vi "Dashboard Main.vi"() -> ()   [LabVIEW 2015]
uses:
  <vilib>/Utility/miscctls.llb/LVRowAndColumnTypeDef.ctl
  <vilib>/event_ctls.llb/eventvkey.ctl
  <vilib>/Rock Robotics/WPI/Dashboard/WPI_DashboardLogging Global.vi
  <vilib>/Utility/config.llb/Write Key (String).vi
  <vilib>/Utility/config.llb/Write Key (I32).vi
  <vilib>/Utility/config.llb/NI_LVConfig.lvlib
  <vilib>/vision/NI_Vision_Development_Module.lvlib
panel:
  in  "TCP":refnum<k5>
  in  "Rec Mode":enum32{"Stop", "Record", "Playback"}(radio)
  in  "Vision":u16(ring)=2 items=["Camera Off", "USB Camera SW", "USB Camera HW", "IP Camera"]
  out "Camera IP":string
  out "Image Message":string="Timeout in Camera Communications"
  in  "Dashboard Tab":T1(tab)
  in  "Two Ball Auto":bool=TRUE
  in  "Defense Selector":u16(ring) items=["Low Bar", "Ramparts", "Moat", "Rock Wall", "Rough Terrain", "Portcullis", "Cheval de Frise", "Drawbridge", "Sally Port"]
  out "Right 2 Current":dbl
  out "Right 1 Current":dbl
  out "Left 2 Current":dbl
  out "Left 1 Current":dbl
  in  "ManipulatorSelector":u16(ring) items=["Portcullis", "Cheval"]
  out "Flip Image":bool
  in  "OK Button":bool
  in  "Position Selector":u16(ring) items=["Far Left", "Pos 2", "Pos 3", "Pos 4", "Far Right"]
  out "NT Connection":bool
  in  "Camera Settings":T2={"Frame Rate"=14, "Compression"=30, "Size"=0} {"Frame Rate" scale=1.0..30.0; "Size" items=["640x480", "320x240", "160x120"]}
  out "Gyro":dbl(knob) scale=0.0..360.0
  out "JS1 Z":dbl(slide) scale=-1.0..1.0 scale format="%#_2e"
  out "JS1 Graph":cluster{"X":dbl, "Y":dbl}[](graph)
  out "JS1 Buttons":T3
  out "JS2 Z":dbl(slide) scale=-1.0..1.0 scale format="%#_2e"
  out "JS2 Graph":cluster{"X":dbl, "Y":dbl}[](graph)
  out "JS2 Buttons":T3
  out "Mode":T4(ring)=enum."Disconnected"
  in  "DB Camera Config":bool
  out "fps":dbl format="%#.1g"
  out "Mbps":dbl=9.6e-05 format="%#.1g"
  out "Mbps LED":bool
  out "Auto Target Enabled":bool
  out "On Target":bool
  out "Ball In Roller":bool
  in  "DB/String 9":string
  in  "DB/String 8":string
  in  "DB/String 7":string
  in  "DB/String 6":string
  in  "DB/String 5":string
  in  "DB/String 4":string
  in  "DB/String 3":string
  in  "DB/String 2":string
  in  "DB/String 1":string
  in  "DB/String 0":string
  in  "DB/Slider 0":dbl(slide) scale=0.0..5.0
  in  "DB/Slider 1":dbl(slide) scale=0.0..5.0
  in  "DB/Slider 2":dbl(slide) scale=0.0..5.0
  in  "DB/Slider 3":dbl(slide) scale=0.0..5.0
  out "DB/LED 3":bool
  out "DB/LED 2":bool
  out "DB/LED 1":bool
  out "DB/LED 0":bool
  in  "DB/Button 3":bool
  in  "DB/Button 2":bool
  in  "DB/Button 1":bool
  in  "DB/Button 0":bool caption="New Name"
  in  "Test Slider":dbl(slide) scale=0.0..100.0 scale format="%#_3g"
  in  "On/Off":bool caption="Solenoid"
  in  "Test Name":u16(ring) items=["Select the test to run..."]
  in  "Test Tree":string(tree)
  in  "Motor":cluster{"Value":dbl, "Enable":bool} {"Value" scale=-1.0..1.0 scale format="%#_3g"}
  out "Progress":T5 {"Test Progress" scale=0.0..100.0}
  in  "Rev/Fwd":cluster{"Forward":bool, "Reverse":bool}
  in  "Test Ring":u16(ring) items=["Monochrome", "Color"]
  out "Cmd Status":string
  in  "Execute Command":bool
  in  "Command Params":string[][](table)
  in  "Command Selection":i32(listbox)
  in  "CheckList":i32(listbox)
  out "Tree":string(tree)
  out "Camera Image":T6(plugin-control)
  out "Background":bool
  # "Left"
  # "Front"
  # "Right"
  # "This tab is a great place for autonomous settings and robot-specific values.\nPlace controls and indicators inside this tab and match name to\nDashboard Variables on robot. You can also delete this comment."
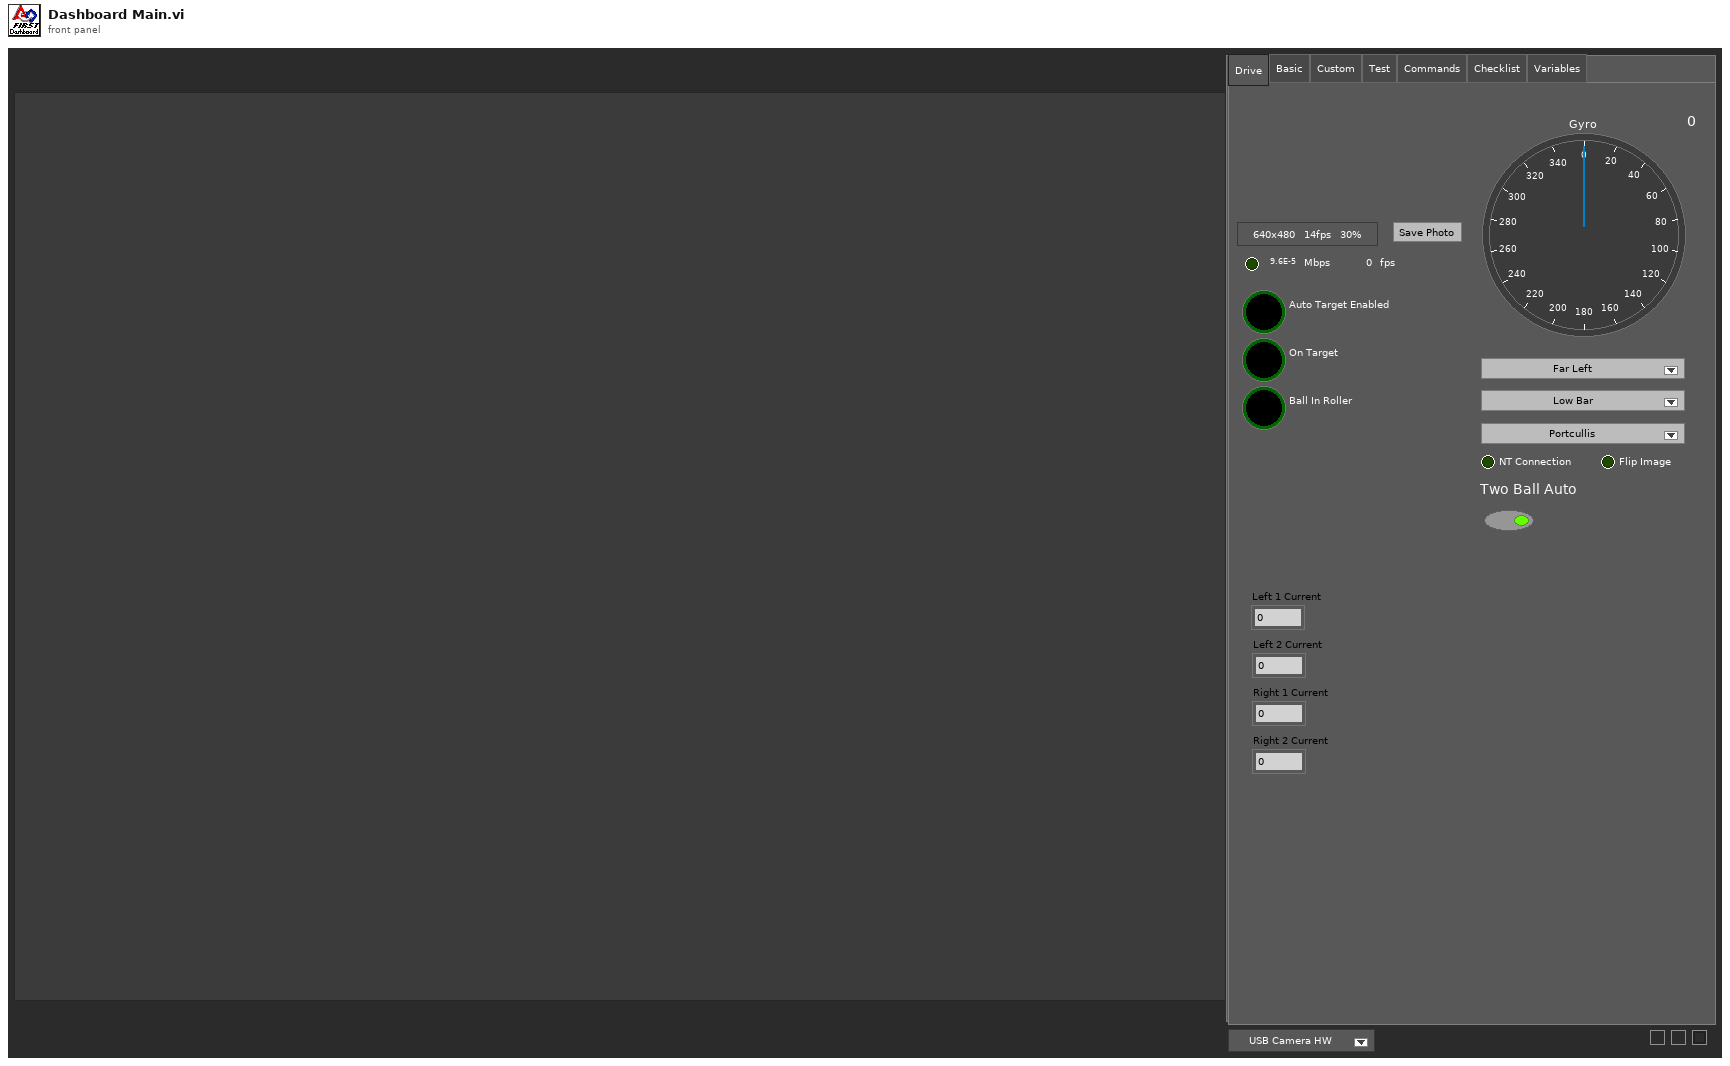
[diagram p1: front panel]
types:
  T1 = enum32{"Drive", "Basic", "Custom", "Test", "Commands", "Checklist", "Variables"}
  T2 = cluster{"Frame Rate":i32, "Compression":i32, "Size":u16}
  T3 = cluster{bool, bool, bool, bool, bool, bool, bool, bool, bool, bool, bool, bool}
  T4 = enum8{"Tele-Op Disabled", "Tele-Op Enabled", "Auto Disabled", "Auto Enabled", "Test Disabled", "Test Enabled", "Disconnected", "No Code", "E-Stop"}
  T5 = cluster{"Test Progress":u8, "Test Progress Text":string}
  T6 = typedef "IMAQ Image.ctl" = refnum<image>
  T7 = typedef "Image Type" = u32
  T8 = cluster{"IDs":cluster{"RPC field ID":u16, "Unique ID":u16}, "String":string}
  T9 = enum32{"Drive", "Basic", "Custom", "Test", "Checklist", "Variables"}
  T10 = cluster{"Camera Image":refnum<vi>, "Dashboard Tab":refnum<vi>, "Background":refnum<vi>, "Vision":refnum<vi>, "Rec Mode":refnum<vi>, "Test Slider":refnum<vi>, "On/Off ":refnum<vi>, "Test Ring":refnum<vi>, "Rev/Fwd":refnum<vi>, "Test Name":refnum<vi>, "Motor":refnum<vi>, "Progress":refnum<vi>, "CheckList":refnum<vi>, "Tree":refnum<vi>, "Test Tree":refnum<vi>, "Command Params":refnum<vi>, "Command Selection":refnum<vi>, "Execute Command":refnum<vi>, "Cmd Status":refnum<vi>}
  T11 = typedef "NI_LVConfig.lvlib/Config Data RefNum.ctl" = refnum<k1>
  T12 = cluster{"Operation":enum16{"Update", "Clear"}, "Color Box":u32}[]
  T13 = typedef "eventvkey.ctl" = enum16{"ASCII", "Enter", "Return", "Shift", "Ctrl", "Alt", "Cmd", "Opt", "Caps", "NumLock", "Clear", "Break", "Up", "Down", "Left", "Right", "Insert", "Delete", "Home", "End", "PageUp", "PageDown", "Escape", "Help", "Pause", "ScrollLock", "F1", "F2", "F3", "F4", "F5", "F6", "F7", "F8", "F9", "F10", "F11", "F12", "F13", "F14", "F15", "F16", "F17", "F18", "F19", "F20", "F21", "F22", "F23", "F24", "Play", "VolumeUp", "VolumeDown", "Mute", "Two Byte Char"}
  T14 = cluster{"Image Size":bool, "Image Type":bool, "Pixel Value":bool, "ROI Information":bool, "Zoom Factor":bool}
  T15 = enum8{"Enabled", "Disabled", "Disabled and Grayed Out"}
  T16 = cluster{"Operation":enum16{"Update", "Clear"}, "Color Box":u32}
  T17 = typedef "LVRowAndColumnTypeDef.ctl" = cluster{"Row":i32, "Column":i32}
  T18 = cluster{"Shift":bool, "Ctrl":bool, "Alt":bool, "Cmd":bool, "Opt":bool}
  T19 = cluster{"Error Strings":string, "Disable Counts":cluster{u16, u16}, "Rail Faults":cluster{u16, u16, u16}, "Robot IP":string, "DB Mode":u8, "Event Info":cluster{"Name":string, "Type":u8, "Number":u16, "Replay":u8}, "Camera Addr":string}
  T20 = cluster{"Storage":cluster{"Disk Free":u64, "RAM Block":u32, "RAM free":u32}, "CPU Utilization":cluster{"CPU % ISR":sgl, "CPU % Time Crit":sgl, "CPU % Timed Str":sgl, "CPU % High":sgl, "CPU % Above":sgl, "CPU % Normal":sgl, "CPU % Low":sgl}, "CAN":cluster{"% Bus Utilization":sgl, "Bus Off Cnt":u32, "TX_FIFO Full Cnt":u32, "Receive Error Cnt":u8, "Transmit Error Cnt":u8}, "HID":cluster{"HID Outputs":u32, "Rumble Low":u16, "Rumble High":u16}[]}
  T21 = cluster{"Status bits":cluster{"Test Mode":bool, "Autonomous":bool, "Enabled":bool, "Code Start":bool, "Brownout":bool, "Reserved 2":bool, "Reserved 3":bool, "E-Stop":bool}, "Code Trace":cluster{"Disabled":bool, "TeleOp":bool, "Auto":bool, "Test":bool}, "Controller Type":enum16{"unknown", "cRIO", "roboRio"}, "Code?":enum16{"unknown", "noCode", "code"}, "Battery V":dbl}
  T22 = cluster{"Control Bits":cluster{"TestMode":bool, "Autonomous":bool, "Enabled":bool, "FMS Present":bool, bool, bool, bool, "E-Stop":bool}, "Team Station ":u8, "Countdown":sgl, "Joystick Values":cluster{"Axes":dbl[], "Buttons":bool[], "POVs":i16[]}[]}
  T23 = cluster{"Axes":dbl[], "Buttons":bool[], "POVs":i16[]}[]
  T24 = cluster{"Axes":dbl[], "Buttons":bool[], "POVs":i16[]}
  T25 = cluster{"Buttons[0]":bool, "Buttons[1]":bool, "Buttons[2]":bool, "Buttons[3]":bool, "Buttons[4]":bool, "Buttons[5]":bool, "Buttons[6]":bool, "Buttons[7]":bool, "Buttons[8]":bool, "Buttons[9]":bool, "Buttons[10]":bool, "Buttons[11]":bool}
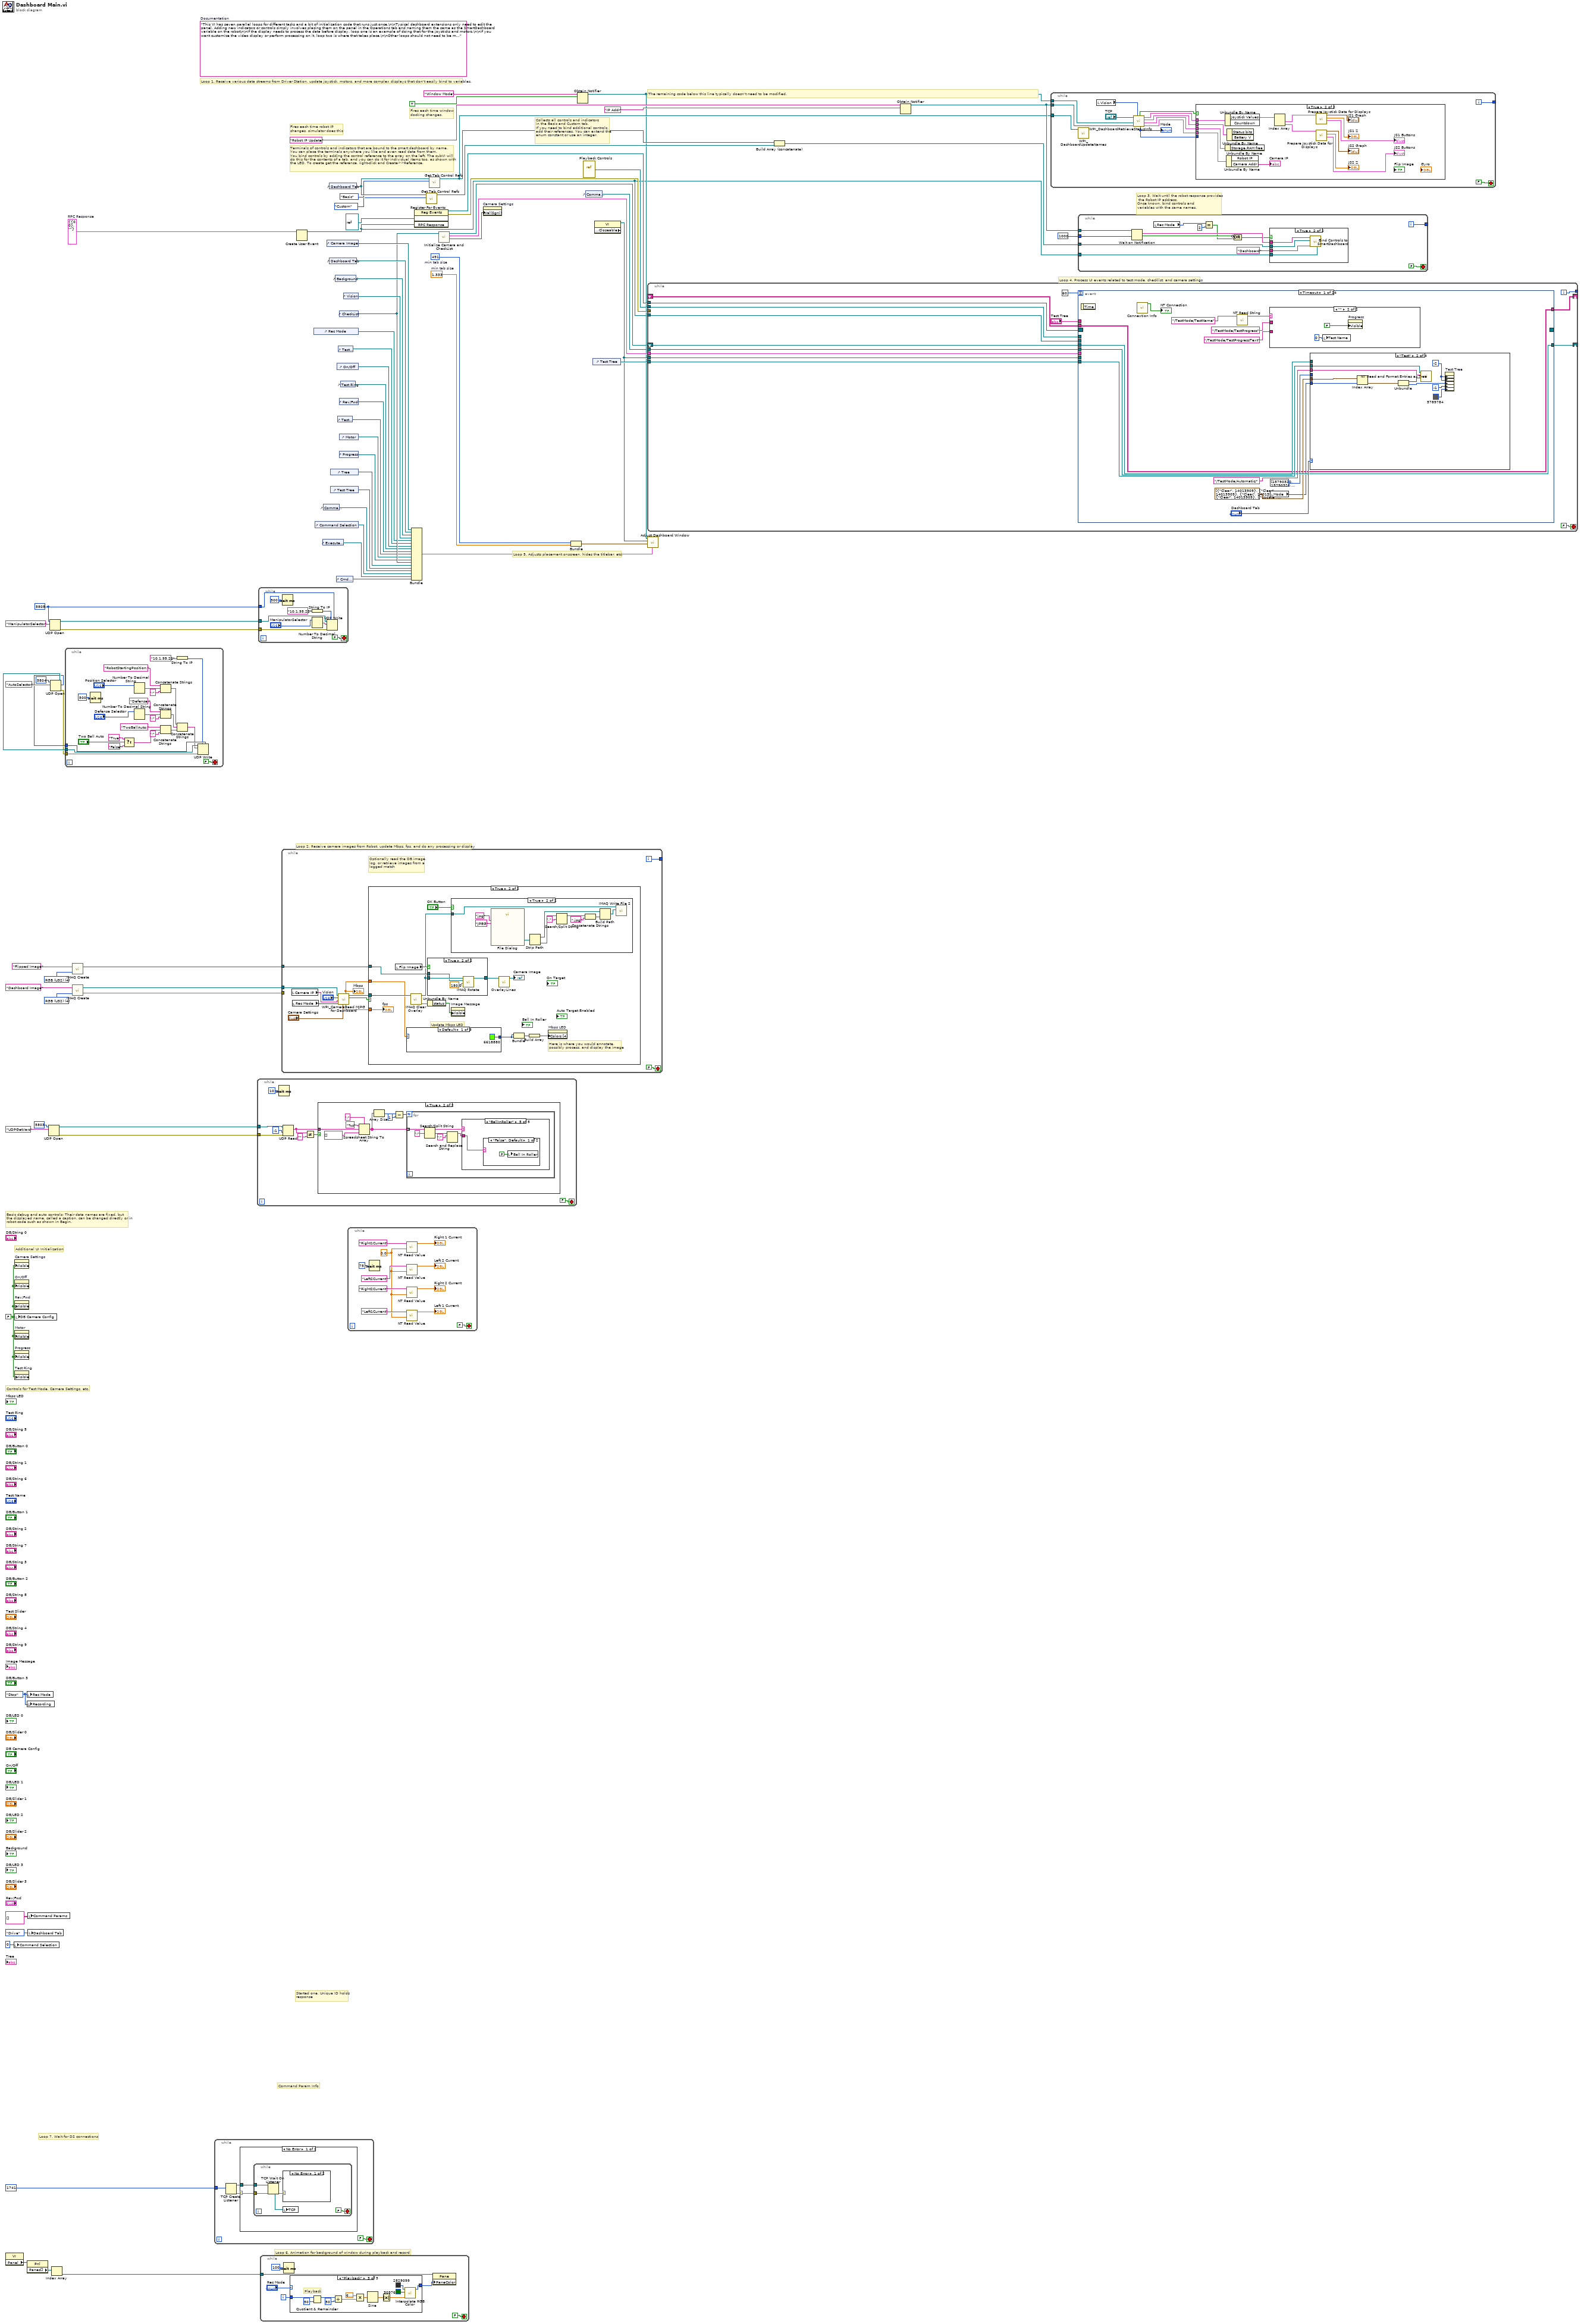
[diagram p0: block diagram]
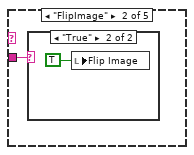
[diagram p4: hidden frame]
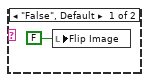
[diagram p5: hidden frame]
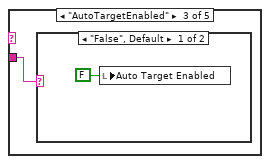
[diagram p6: hidden frame]
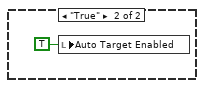
[diagram p7: hidden frame]
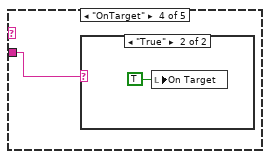
[diagram p8: hidden frame]
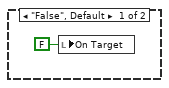
[diagram p9: hidden frame]
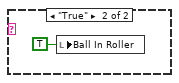
[diagram p10: hidden frame]
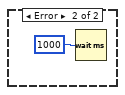
[diagram p11: hidden frame]
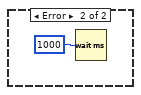
[diagram p12: hidden frame]
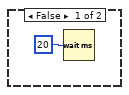
[diagram p13: hidden frame]
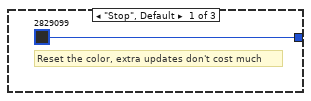
[diagram p14: hidden frame]
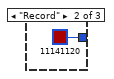
[diagram p15: hidden frame]
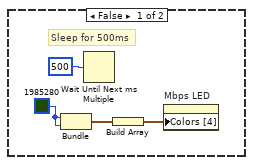
[diagram p17: hidden frame]
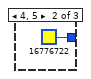
[diagram p20: hidden frame]
diagram:
  w1 = u16 5805 ("port")
  w7 = T7 4 items=["Grayscale (U8)", "Grayscale (I16)", "Grayscale (SGL)", "Complex (CSG)", "RGB (U32)", "HSL (U32)", "RGB (U64)"] ("Image Type")
  w23 = T8 {"IDs"={"RPC field ID"=0, "Unique ID"=0}, "String"=""}  # RPC Response
  w49 = 491  # min tab size
  w48 = 1.333  # min tab size
  w57 = enum32{"Stop", "Record", "Playback"}."Stop" ("Rec Mode")
  w31 = FALSE ("Visible")
  (unwired) "This VI has seven parallel loops for different tasks and a bit of initialization code that runs just once.\n\nTypical dashboard extensions only need to edit the panel. Adding new indicators or controls simply involves placing them on the panel in the Operations tab and naming them the same as the SmartDashboard variable on the robot\n\nIf the display needs to process the data before display, loop one is an example of doing that for the joysticks and motors.\n\nIf you want customize the video display or perform processing on it, loop two is where that takes place.\n\nOther loops should not need to be modified. They are pretty standard, and document the task they perform."  # Documentation
  w77 = T7 4 items=["Grayscale (U8)", "Grayscale (I16)", "Grayscale (SGL)", "Complex (CSG)", "RGB (U32)", "HSL (U32)", "RGB (U64)"] ("Image Type")
  # "Command Param Info"
  # "Started one, Unique ID holds\nresponse"
  # "Loop 7. Wait for DS connections"
  # "Basic debug and auto controls: Their data names are fixed, but\nthe displayed name, called a caption, can be changed directly or in\nrobot code such as shown in Begin."
  # "Controls for Test Mode, Camera Settings, etc."
  # "Additional UI Initialization"
  # "Loop 6. Animation for background of window during playback and record"
  # "Fires each time robot IP\nchanges, simulator does this"
  # "Fires each time window\ndocking changes."
  # "Collects all controls and indicators\nin the Basic and Custom tab.\nIf you need to bind additional controls,\nadd their references. You can extend the\nenum constant or use an integer."
  # "The remaining code below this line typically doesn't need to be modified."
  # "Loop 4. Process UI events related to test mode, checklist, and camera settings"
  # "Terminals of controls and indicators that are bound to the smart dashboard by name.\nYou can place the terminals anywhere you like and even read data from them.\nYou bind controls by adding the control reference to the array on the left. The subVI will\ndo this for the contents of a tab, and you can do it for individual items too, as shown with\nthe LED. To create get the reference, right-click and Create>>Reference."
  # "Loop 3. Wait until the robot response provides\n the Robot IP address.\nOnce known, bind controls and\nvariables with the same names."
  # "Loop 5. Adjusts placement onscreen, hides the titlebar, etc."
  # "Loop 1. Receive various data streams from Driver Station, update joystick, motors, and more complex displays that don't easily bind to variables."
  # "Loop 2. Receive camera images from Robot, update Mbps, fps, and do any processing or display"
  n1 = property class="VI"() -> ("Panel"=w64:refnum<vi>)  [unwired: 2 in, 2 out]
  n2 = local write "Command Selection"(u16 0 ("milliseconds to wait")) -> ()
  n3 = property on="Camera Settings" class="Clust (strict)"("Visible"=w31) -> ()  [unwired: 2 in, 2 out]
  n4 = property on="On/Off" class="Bool (strict)"("Visible"=w31) -> ()  [unwired: 2 in, 2 out]
  n5 = property on="Rev/Fwd" class="Clust (strict)"("Visible"=w31) -> ()  [unwired: 2 in, 2 out]
  n6 = local write "DB Camera Config"(w31) -> ()
  n7 = property on="Motor" class="Clust (strict)"("Visible"=w31) -> ()  [unwired: 2 in, 2 out]
  n8 = property on="Progress" class="Clust (strict)"("Visible"=w31) -> ()  [unwired: 2 in, 2 out]
  n9 = property on="Test Ring" class="Ring (strict)"("Visible"=w31) -> ()  [unwired: 2 in, 2 out]
  n10 = local write "Rec Mode"(w57) -> ()
  n11 = global write "WPI_DashboardLogging Global.vi" "Recording"(w57) -> ()
  n12 = property class="Pnl"(reference=w64) -> ("Panes[]"=w65:refnum<vi>[])  [unwired: 1 in, 2 out]
  n13 = local write "Command Params"(string[][] [] ("Command Params")) -> ()
  n14 = local write "Dashboard Tab"(T1."Drive" ("Dashboard Tab")) -> ()
  n15 = UDP Open(10:"UDPGetVars" ("service name"), 11:u16 5803 ("port")) -> (port=w11:refnum<k16>, 0:w10:errorcluster)  [unwired: 3 in, 1 out]
  n16 = UDP Open(10:"ManipulatorSelector" ("service name"), 11:w1) -> (port=w4:refnum<k16>, 0:w3:errorcluster)  [unwired: 3 in, 1 out]
  n17 = UDP Open(10:"AutoSelector" ("service name"), 11:u16 5804 ("port")) -> (port=w14:refnum<k16>, 0:w12:errorcluster, 2:w13:u16)  [unwired: 3 in]
  n18 = Index Array(array=w65) -> (element=w63:refnum<vi>)  [unwired: 1 in]
  n19 = while {
    tunnel: w14 -> [w100]
    tunnel: w13 -> [w99]
    tunnel: w12 -> [w96]
    stop <- FALSE stop-if-true
    n20 = Wait (ms)(milliseconds to wait=u32 500) -> ()  [unwired: 1 out]
    n21 = Select(t="True" ("string"), s="Two Ball Auto", f="False" ("string")) -> (s? t:f=w81:string)
    n22 = Number To Decimal String(number="Position Selector") -> (decimal integer string=w94:string)  [unwired: 1 in]
    n23 = Number To Decimal String(number="Defense Selector") -> (decimal integer string=w90:string)  [unwired: 1 in]
    n24 = Concatenate Strings("RobotStartingPosition:" ("string"), w94, ";" ("string")) -> (w85:string)
    n25 = Concatenate Strings("Defense:" ("string"), w90, ";" ("string")) -> (w84:string)
    n26 = Concatenate Strings("TwoBallAuto:" ("string"), w81, ";" ("string")) -> (w82:string)
    n27 = String To IP(1:"10.1.95.22") -> (0:w97:u32)
    n28 = Concatenate Strings(w85, w84, w82) -> (w83:string)
    n29 = UDP Write(address=w97, port or service name=w99, connection ID=w100, data in=w83, 8:w96) -> ()  [unwired: 1 in, 2 out]
  }
  n30 = call "IMAQ Create"("Image Name"="Flipped Image", "Image Type"=w7) -> ("New Image"=w5:T6)  [unwired: 2 in, 2 out]
  n31 = call "IMAQ Create"("Image Name"="Dashboard Image", "Image Type"=w77) -> ("New Image"=w75:T6, "error out"=w74:errorcluster)  [unwired: 2 in, 1 out]
  n32 = while {
    tunnel: u16 1741 ("timeout ms (25000)") -> [w104]
    stop <- FALSE stop-if-true
    n33 = TCP Create Listener(10:w104) -> (0:w103:errorcluster, 3:w105:refnum<k5>)  [unwired: 4 in, 1 out]
    n34 = case shown="No Error" w103 {
      selector: w103 -> [w107 _]
      tunnel: w105 -> [w108 _]
      frame No Error {
        n35 = while {
          tunnel: w108 -> [w111]
          tunnel: w107 -> [w110]
          stop <- FALSE stop-if-true
          n36 = TCP Wait On Listener(8:w110, 11:w111) -> (0:w112:errorcluster, 4:w113:refnum<k5>)  [unwired: 2 in, 3 out]
          n37 = case shown="No Error" w112 {
            frame No Error {
            }
            frame Error {
              n38 = Wait (ms)(milliseconds to wait=u32 1000) -> ()  [unwired: 1 out]
            }
          }
          n39 = local write "TCP"(w113) -> ()
        }
      }
      frame Error {
        n40 = Wait (ms)(milliseconds to wait=u32 1000) -> ()  [unwired: 1 out]
      }
    }
  }
  n41 = while {
    tunnel: w11 -> [w120]
    tunnel: w10 -> [w119]
    stop <- FALSE stop-if-true
    n42 = Wait (ms)(milliseconds to wait=u32 10) -> ()  [unwired: 1 out]
    n43 = UDP Read(connection ID=w120, timeout ms (25000)=-1, 8:w119) -> (data out=w116:string)  [unwired: 1 in, 4 out]
    n44 = Not Equal?(x=w116, y="") -> (x != y?=w117:bool)
    n45 = case shown="True" w117 {
      tunnel: w116 -> [_ w131]
      frame False {
      }
      frame True {
        n46 = Spreadsheet String To Array(delimiter (Tab)=";" ("search string/char (-)"), format string="%s", spreadsheet string=w131, array type (2D Dbl)=string[] []) -> (array=w127:string[])
        n47 = Array Size(array=w127) -> (size(s)=w126:i32)
        n48 = Subtract(x=w126, y=1) -> (x-y=w124:i32)
        n49 = for {
          N: w124 -> [_]
          tunnel: w127 -> [w137] mode=indexing
          n50 = Search/Split String(string=w137, search string/char (-)=":") -> (substring before match=w135:string, match + rest of string=w134:string)  [unwired: 1 in, 1 out]
          n51 = Search and Replace String(input string=w134, search string=":" ("replace string (\"\")")) -> (result string=w132:string)  [unwired: 6 in, 3 out]
          n52 = case shown="\"BallInRoller\"" w135 {
            tunnel: w132 -> [_ w138 w141 w144 w147]
            frame "False", Default {
            }
            frame "FlipImage" {
              n53 = case shown="\"True\"" w138 {
                frame "False", Default {
                  n54 = local write "Flip Image"(FALSE ("Flip Image")) -> ()
                }
                frame "True" {
                  n55 = local write "Flip Image"(TRUE ("Flip Image")) -> ()
                }
              }
            }
            frame "AutoTargetEnabled" {
              n56 = case shown="\"False\", Default" w141 {
                frame "False", Default {
                  n57 = local write "Auto Target Enabled"(FALSE ("Auto Target Enabled")) -> ()
                }
                frame "True" {
                  n58 = local write "Auto Target Enabled"(TRUE ("Auto Target Enabled")) -> ()
                }
              }
            }
            frame "OnTarget" {
              n59 = case shown="\"True\"" w144 {
                frame "False", Default {
                  n60 = local write "On Target"(FALSE ("On Target")) -> ()
                }
                frame "True" {
                  n61 = local write "On Target"(TRUE ("On Target")) -> ()
                }
              }
            }
            frame "BallInRoller" {
              n62 = case shown="\"False\", Default" w147 {
                frame "False", Default {
                  n63 = local write "Ball In Roller"(FALSE ("Ball In Roller")) -> ()
                }
                frame "True" {
                  n64 = local write "Ball In Roller"(TRUE ("Ball In Roller")) -> ()
                }
              }
            }
          }
        }
      }
    }
  }
  n65 = while {
    tunnel: w4 -> [w152]
    tunnel: w3 -> [w151]
    tunnel: w1 -> [w150]
    stop <- FALSE stop-if-true
    n66 = Wait (ms)(milliseconds to wait=u32 500) -> ()  [unwired: 1 out]
    n67 = String To IP(1:"10.1.95.22") -> (0:w156:u32)
    n68 = Number To Decimal String(number="ManipulatorSelector") -> (decimal integer string=w157:string)  [unwired: 1 in]
    n69 = UDP Write(address=w156, port or service name=w150, connection ID=w152, data in=w157, 8:w151) -> ()  [unwired: 1 in, 2 out]
  }
  n70 = while {
    tunnel: w63 -> [w160]
    i -> [w163]
    stop <- FALSE stop-if-true
    n71 = Wait (ms)(milliseconds to wait=u32 100) -> ()  [unwired: 1 out]
    n72 = case shown="\"Playback\"" "Rec Mode" {
      tunnel: w163 -> [_ _ w178]
      tunnel: [u32 2829099 ("Base Color") u32 11141120 ("Target Color") w167] -> w159
      frame "Stop", Default {
        # "Reset the color, extra updates don't cost much"
      }
      frame "Record" {
      }
      frame "Playback" {
        # "Playback"
        n73 = Quotient & Remainder(x=w178, y=u32 50 ("milliseconds to wait")) -> (x-y*floor(x/y)=w174:u32)  [unwired: 1 out]
        n74 = Divide(x=w174, y=u32 50 ("milliseconds to wait")) -> (x/y=w171:dbl)
        n75 = Multiply(x=6.283185307179586, y=w171) -> (x*y=w176:dbl)
        n76 = Sine(x=w176) -> (sin(x)=w175:dbl)
        n77 = Absolute Value(x=w175) -> (abs(x)=w168:dbl)
        n78 = call "Interpolate RGB Color.vi"("Proportion"=w168, "Target Color"=u32 30976, "Base Color"=u32 2829099) -> ("Result Color"=w167:u32)  [unwired: 8 in]
      }
    }
    n79 = property class="Pane"(reference=w160, "PaneColor"=w159) -> ()  [unwired: 1 in, 2 out]
  }
  n80 = while {
    tunnel: w75 -> [w188]
    tunnel: w74 -> [_]
    tunnel: [w189] -> _
    tunnel: w5 -> [w179]
    i -> [w189]
    stop <- FALSE stop-if-true
    # "Optionally read the DB image,\nlog, or retrieve images from a\nlogged match"
    n81 = local read "Camera IP"() -> (w181:string)
    n82 = local read "Rec Mode"() -> (w183:enum32{"Stop", "Record", "Playback"})
    n83 = call <vilib>:"WPI_CameraRead MJPG for Dashboard.vi"("Camera Settings"="Camera Settings", "Rec Mode"=w183, "Camera IP"=w181, "Camera Mode"="Vision", "Refnum in"=w188) -> ("Active"=w186:bool, "Refnum out"=w187:T6, "FPS"=w185:dbl, "Bandwidth (Mbps)"=w180:dbl)  [unwired: 3 in]
    "Mbps" <- w180
    n84 = case shown="True" w186 {
      tunnel: w187 -> [_ w203]
      tunnel: w180 -> [_ w202]
      tunnel: w185 -> [_ w201]
      tunnel: w179 -> [_ w199]
      frame False {
        w191 = u32 1985280 ("Color Box")
        # "Sleep for 500ms"
        n85 = Bundle("Color Box"=w191, "Color Box"=w191) -> (w193:cluster{"Color Box":u32, "Color Box":u32})  [unwired: 1 out]
        n86 = Wait Until Next ms Multiple(millisecond multiple=u32 500) -> ()  [unwired: 1 out]
        n87 = Build Array(w193) -> (w192:cluster{"Color Box":u32, "Color Box":u32}[])
        n88 = property on="Mbps LED" class="Bool (strict)"("Colors [4]"=w192) -> ()  [unwired: 2 in, 2 out]
      }
      frame True {
        # "Here is where you would annotate,\npossibly process, and display the image"
        # "Update Mbps LED"
        n89 = local read "Flip Image"() -> (w198:bool)
        n90 = case shown="Default" w202 {
          tunnel: [u32 6618880 ("Color Box") u32 16776722 ("Color Box") u32 16716800 ("Color Box")] -> w204
          frame Default {
          }
          frame 4, 5 {
          }
          frame 6.. {
          }
        }
        n91 = call "IMAQ Clear Overlay"("Image"=w203) -> ("error out"=w207:errorcluster, "Image Out"=w195:T6)  [unwired: 2 in, 7 out]
        n92 = case shown="True" w198 {
          tunnel: w195 -> [w209 w213]
          tunnel: w199 -> [_ w212]
          tunnel: [w209 w210] -> w197
          frame False {
          }
          frame True {
            n93 = call "IMAQ Rotate"("Angle (degrees)"=sgl 180.0, "Image Dst"=w212, "Image Src"=w213) -> ("Image Dst Out"=w210:T6)  [unwired: 7 in, 1 out]
          }
        }
        n94 = Unbundle By Name(w207) -> ("status"=w208:bool)
        n95 = case shown="True" "OK Button" {
          tunnel: w195 -> [_ w214]
          frame False {
          }
          frame True {
            n96 = call "File Dialog"("pattern (all files)"="jpg", "pattern label"="JPEG") -> ("selected path"=w222:path)  [unwired: 10 in, 3 out]
            n97 = Strip Path(path=w222) -> (stripped path=w221:path, name=w220:string)
            n98 = Search/Split String(string=w220, search string/char (-)=".") -> (substring before match=w218:string)  [unwired: 1 in, 2 out]
            n99 = Concatenate Strings(w218, ".jpg" ("string")) -> (w216:string)
            n100 = Build Path(base path=w221, name or relative path=w216) -> (appended path=w215:path)
            n101 = call-poly "IMAQ Write File 2"("File Path"=w215, "Image"=w214) -> ()  [unwired: 8 in, 2 out]
          }
        }
        n102 = property on="Image Message" class="Str"("Visible"=w208) -> ()  [unwired: 2 in, 2 out]
        n103 = call "OverlayLines.vi"("Image"=w197) -> ("Image Out"=→"Camera Image":T6)  [unwired: 10 in]
        n104 = Bundle("Color Box"=w204, "Color Box"=w204) -> (w206:cluster{"Color Box":u32, "Color Box":u32})  [unwired: 1 out]
        n105 = Build Array(w206) -> (w205:cluster{"Color Box":u32, "Color Box":u32}[])
        n106 = property on="Mbps LED" class="Bool (strict)"("Colors [4]"=w205) -> ()  [unwired: 2 in, 2 out]
        "fps" <- w201
      }
    }
  }
  n107 = Create User Event(user event datatype=w23) -> (user event=w19:refnum<user-event>)  [unwired: 1 in, 1 out]
  n108 = control-ref of="Rec Mode"() -> (w37:refnum<vi>)
  n109 = control-ref of="Command Selection"() -> (w22:refnum<vi>)
  n110 = control-ref of="Execute Command"() -> (w24:refnum<vi>)
  n111 = control-ref of="Command Params"() -> (w25:refnum<vi>)
  n112 = control-ref of="Camera Image"() -> (w52:refnum<vi>)
  n113 = control-ref of="Dashboard Tab"() -> (w55:refnum<vi>)
  n114 = control-ref of="Dashboard Tab"() -> (w51:refnum<vi>)
  n115 = control-ref of="Tree"() -> (w41:refnum<vi>)
  n116 = control-ref of="Test Tree"() -> (w40:refnum<vi>)
  n117 = control-ref of="Background"() -> (w46:refnum<vi>)
  n118 = control-ref of="Cmd Status"() -> (w18:refnum<vi>)
  n119 = control-ref of="On/Off"() -> (w35:refnum<vi>)
  n120 = control-ref of="Test Name"() -> (w39:refnum<vi>)
  n121 = control-ref of="Test Slider"() -> (w36:refnum<vi>)
  n122 = control-ref of="CheckList"() -> (w42:refnum<vi>)
  n123 = control-ref of="Rev/Fwd"() -> (w33:refnum<vi>)
  n124 = control-ref of="Motor"() -> (w38:refnum<vi>)
  n125 = control-ref of="Progress"() -> (w32:refnum<vi>)
  n126 = control-ref of="Test Ring"() -> (w34:refnum<vi>)
  n127 = control-ref of="Vision"() -> (w50:refnum<vi>)
  n128 = while {
    stop <- FALSE stop-if-true
    w231 = 0.0 ("Default Value")
    n129 = Wait (ms)(milliseconds to wait=u32 75) -> ()  [unwired: 1 out]
    n130 = call-poly <vilib>:"NT Read Value.vi"("Default Value"=w231, "Name"="Right1Current") -> ("Numeric"=→"Right 1 Current":dbl)  [unwired: 8 in, 1 out]
    n131 = call-poly <vilib>:"NT Read Value.vi"("Default Value"=w231, "Name"="Left2Current") -> ("Numeric"=→"Left 2 Current":dbl)  [unwired: 8 in, 1 out]
    n132 = call-poly <vilib>:"NT Read Value.vi"("Default Value"=w231, "Name"="Right2Current") -> ("Numeric"=→"Right 2 Current":dbl)  [unwired: 8 in, 1 out]
    n133 = call-poly <vilib>:"NT Read Value.vi"("Default Value"=w231, "Name"="Left1Current") -> ("Numeric"=→"Left 1 Current":dbl)  [unwired: 8 in, 1 out]
  }
  n134 = Bundle("Camera Image"=w52, "Dashboard Tab"=w51, "Background"=w46, "Vision"=w50, "Rec Mode"=w37, "Test Slider"=w36, "On/Off"=w35, "Test Ring"=w34, "Rev/Fwd"=w33, "Test Name"=w39, "Motor"=w38, "Progress"=w32, "CheckList"=w42, "Tree"=w41, "Test Tree"=w40, "Command Params"=w25, "Command Selection"=w22, "Execute Command"=w24, "Cmd Status"=w18) -> (w43:T10)  [unwired: 1 in]
  n135 = register-events(refnum<vi> refnum, w19) -> (reference out=w61:refnum<event-registration>, error out=w60:errorcluster)  [unwired: 2 in]
  n136 = call <vilib>:"Get Tab Control Refs.vi"("Page Index"=T9."Custom" ("Dashboard Tab"), "TabControl in"=w55) -> ("ControlsOnPage"=w54:refnum<vi>[])  [unwired: 9 in]
  n137 = call <vilib>:"Get Tab Control Refs.vi"("Page Index"=T9."Basic" ("Dashboard Tab"), "TabControl in"=w55) -> ("ControlsOnPage"=w29:refnum<vi>[])  [unwired: 9 in]
  n138 = call "Initialize Camera and CheckList.vi"("ListBox in"=w42) -> ("Cluster"=w68:cluster{"value":i32, "value":i32, "index":i32}, "Array"=w69:cluster{string[]}[], "File Refnum"=w67:T11)  [unwired: 8 in]
  n139 = property on="Camera Settings" class="Clust (strict)"("Val(Sgnl)"=w68) -> ()  [unwired: 2 in, 2 out]
  n140 = Bundle("min tab size"=w49, "min tab size"=w48) -> (w47:cluster{"min tab size":i32, "min tab size":dbl})  [unwired: 1 in]
  n141 = Obtain Notifier(name (unnamed)="Window Mode", notification data type=TRUE) -> (notifier out=w28:refnum<notifier>)  [unwired: 2 in, 2 out]
  n142 = vi-ref "Playback Controls.vi"() -> (w62:refnum<vi>)
  n143 = control-ref of="Command Params"() -> (w17:refnum<vi>)
  n144 = control-ref of="Test Tree"() -> (w66:refnum<vi>)
  n145 = property class="VI" props=["Front Panel.Closeable"]() -> (reference out=w56:refnum<vi>)  [unwired: 2 in, 2 out]
  n146 = while {
    tunnel: w69 -> [w250]
    shift-right: [w249] -> _
    shift-left: w67 -> [w248]
    tunnel: [w247] -> _
    tunnel: w66 -> [w246]
    tunnel: w62 -> [w245]
    tunnel: w61 -> [w244]
    tunnel: w60 -> [_]
    tunnel: w56 -> [w243]
    tunnel: w19 -> [w242]
    tunnel: w17 -> [w241]
    shift-right: [w240] -> _
    shift-left: _ -> [w239]
    i -> [w247]
    stop <- FALSE stop-if-true
    n147 = event shown="[0] Timeout" {
      selector: w244 -> [_ _ _ _ _ _ _ _ _ _ _ _ _ _ _ _ _ _ _ _ _ _ _ _]
      dyn-events: [_ _ _ _ _ _ _ _ _ _ _ _ _ _ _ _ _ _ w557 _ _ _ _ _] -> _
      timeout: u32 60 ("milliseconds to wait") -> [_ _ _ _ _ _ _ _ _ _ _ _ _ _ _ _ _ _ _ _ _ _ _ _]
      tunnel: w246 -> [w263 _ _ _ _ _ _ _ _ _ _ _ _ _ _ _ _ _ _ _ _ _ _ _]
      tunnel: "Test Tree" -> [_ _ _ _ _ _ _ _ _ _ _ _ _ w520 w529 w532 w537 w546 _ _ _ _ _ _]
      tunnel: w250 -> [_ w301 _ _ _ _ _ _ _ _ _ w482 w513 _ _ _ _ _ _ _ _ _ _ _]
      tunnel: [w260 w300 w404 w410 w419 w422 w428 w440 w448 w454 w467 w481 w506 w519 w527 w531 w536 w545 w559 w575 w577 w585 w596 w601] -> w249
      tunnel: w248 -> [w260 w300 w404 w410 w419 w422 w428 w440 w448 w454 w467 w480 w506 w519 w527 w531 w536 w545 w559 w575 w577 w585 w596 w601]
      tunnel: w245 -> [_ _ _ _ _ _ _ _ _ _ _ _ _ _ _ _ _ _ w560 _ w580 _ _ _]
      tunnel: w243 -> [_ _ _ _ _ _ _ _ _ _ _ _ _ _ _ _ _ _ w555 _ _ _ _ _]
      tunnel: w242 -> [_ _ _ _ _ _ _ _ _ _ _ _ _ _ _ _ _ _ w551 _ _ _ _ _]
      tunnel: w241 -> [w255 _ _ _ _ _ w426 _ _ _ _ _ _ _ _ _ _ _ _ _ _ _ _ _]
      tunnel: [w254 w299 w403 w409 w418 w423 w424 w434 w445 w453 w466 w479 w505 w518 w526 w530 w535 w544 w550 w573 w576 w581 w589 w602] -> w240
      tunnel: w239 -> [w254 w299 w403 w409 w418 w423 w424 _ _ w453 w466 w479 w505 w518 w526 w530 w535 w544 w550 w573 w576 w581 w589 w602]
      event Timeout {
        n148 = event-data() -> ()  [unwired: 1 in, 1 out]
        n149 = call <vilib>:"Connextion Info.vi"() -> ("Connected"=→"NT Connection":bool)  [unwired: 10 in, 1 out]
        n150 = call <vilib>:"NT Read String.vi"("Name"="/TestMode/TestName") -> ("String"=w266:string)  [unwired: 9 in, 1 out]
        n151 = case shown="\"\"" w266 {
          tunnel: "/TestMode/TestProgress" ("Name") -> [w293 _]
          tunnel: "/TestMode/TestProgressText" ("Name") -> [w292 _]
          frame Default {
            n152 = call <vilib>:"NT Read Number.vi"("Name"=w293) -> ("Numeric"=w294:dbl)  [unwired: 9 in, 1 out]
            n153 = call <vilib>:"NT Read String.vi"("Name"=w292) -> ("String"=w295:string)  [unwired: 9 in, 1 out]
            n154 = Bundle("Numeric"=w294, "String"=w295) -> (→"Progress":cluster{"Numeric":dbl, "String":string})  [unwired: 1 in]
          }
          frame "" {
            n155 = local write "Test Name"(u16 0) -> ()
            n156 = property on="Progress" class="Clust (strict)"("Visible"=FALSE) -> ()  [unwired: 2 in, 2 out]
          }
        }
        n157 = local read "Mode"() -> (w257:T4)
        n158 = case shown="\"Test\"" "Dashboard Tab" {
          tunnel: w263 -> [_ w277 _ _]
          tunnel: "/TestMode/Automatic/" ("Name Pattern") -> [_ w276 _ _]
          tunnel: T12 [{"Operation"=enum."Clear", "Color Box"=14013909}, {"Operation"=enum."Clear", "Color Box"=14013909}, {"Operation"=enum."Clear", "Color Box"=14013909}, {"Operation"=enum."Clear", "Color Box"=14013909}, {"Operation"=enum."Update", "Color Box"=14013909}, {"Operation"=enum."Update", "Color Box"=16777215}, {"Operation"=enum."Clear", "Color Box"=14013909}, {"Operation"=enum."Clear", "Color Box"=14013909}, {"Operation"=enum."Clear", "Color Box"=14013909}] -> [_ w269 _ w286]
          tunnel: w257 -> [_ w268 _ w285]
          tunnel: u32[] [15790320, 15790320, 15790320, 15790320, 16777215, 16777215, 15790320, 15790320, 15790320] -> [_ _ _ w291]
          tunnel: w255 -> [_ _ _ w279]
          frame "Custom", Default {
          }
          frame "Test" {
            w275 = -2 ("Active Item:Row Number")
            n159 = Index Array(array=w269, index=w268) -> (element=w270:T16)
            n160 = Unbundle(w270) -> ("Operation"=w271:enum16{"Update", "Clear"}, "Color Box"=w272:u32)
            n161 = call <vilib>:"NT Read and Format Entries as Tree.vi"("Operation"=w271, "Name Pattern"=w276, "Tree Refnum"=w277) -> ()  [unwired: 7 in, 2 out]
            n162 = property on="Test Tree" class="Tree (strict)"("Active Item Row Number"=w275, "ActiveColNum"=w275, "CellBG"=w272, "Active Item Row Number"=-1 ("Active Item:Row Number"), "CellBG"=u32 5789784 ("Color Box")) -> ()  [unwired: 2 in, 2 out]
          }
          frame "Variables" {
            n163 = control-ref of="Tree"() -> (w278:refnum<vi>)
            n164 = call <vilib>:"NT Read and Format Entries as Tree.vi"("Tree Refnum"=w278) -> ()  [unwired: 9 in, 2 out]
          }
          frame "Commands" {
            w287 = u32 5789784 ("Color Box")
            w288 = T17 {"Row"=-1, "Column"=-2} ("Active Cell:Active Cell")
            w290 = T17 {"Row"=-2, "Column"=-2} ("Active Cell:Active Cell")
            n165 = Index Array(array=w286, index=w285) -> (element=w284:T16)
            n166 = Index Array(array=w291, index=w285) -> (element=w289:u32)
            n167 = property on="Command Selection" class="MCListbox (strict)"("ActiveCell"=w290, "CellBG"=w289, "ActiveCell"=w288, "CellBG"=w287) -> ()  [unwired: 2 in, 2 out]
            n168 = property on="Command Params" class="Tbl (strict)"("Active Cell"=w290, "Cell BG Color"=w289, "Active Cell"=w288, "Cell BG Color"=w287) -> ()  [unwired: 2 in, 2 out]
            n169 = Unbundle(w284) -> ("Operation"=w283:enum16{"Update", "Clear"})  [unwired: 1 out]
            n170 = local read "Command Selection"() -> (w282:i32)
            n171 = call <vilib>:"WPI_DashboardUpdate RPC Info.vi"("Operation"=w283) -> ("update"=w281:bool, "commands"=w280:string[][])  [unwired: 9 in]
            n172 = property on="Command Selection" class="MCListbox (strict)"("ItemNames"=w280) -> ()  [unwired: 2 in, 2 out]
            n173 = call <vilib>:"WPI_DashboardUpdate Command Params.vi"("Update"=w281, "NewVal"=w282, "Commands"=w280, "Param Tbl"=w279) -> ()  [unwired: 7 in, 1 out]
          }
        }
      }
      event "Test Tree": Value Change {
        # "Show appropriate\ncontrols"
        n174 = event-data() -> ("CtlRef"=w304:refnum<vi>, "NewVal"=w302:string)  [unwired: 1 in]
        n175 = property on="Progress" class="Clust (strict)"("Visible"=FALSE) -> ()  [unwired: 2 in, 2 out]
        n176 = call <vilib>:"WPI_UtilitiesGetTreeIOName.vi"("NewVal"=w302, "TreeControl in"=w304) -> ("I/O Name"=w305:string)  [unwired: 9 in]
        n177 = case shown="\"Analog Out\", \"Motor\", \"PWM\"" w305 {
          selector: w305 -> [_ w312 _ w334 w343 _]
          tunnel: w302 -> [_ _ w331 w333 _ w350]
          tunnel: w301 -> [_ _ _ _ _ w349]
          frame Default {
            w307 = FALSE ("Visible")
            w306 = FALSE ("Visible")
            n178 = property on="Test Ring" class="Ring (strict)"("Visible"=w306) -> ()  [unwired: 2 in, 2 out]
            n179 = property on="Motor" class="Clust (strict)"("Visible"=w306) -> ()  [unwired: 2 in, 2 out]
            n180 = property on="Test Slider" class="Slide (strict)"("Visible"=w307) -> ()  [unwired: 2 in, 2 out]
            n181 = property on="On/Off" class="Bool (strict)"("Visible"=w307) -> ()  [unwired: 2 in, 2 out]
            n182 = property on="Rev/Fwd" class="Clust (strict)"("Visible"=w307) -> ()  [unwired: 2 in, 2 out]
          }
          frame "Analog Out", "Motor", "PWM" {
            w313 = FALSE ("Visible")
            n183 = case shown="\"Analog Out\"" w312 {
              tunnel: [1.0 ("Value") -1.0 ("Value") 0.0 ("Value")] -> w311
              tunnel: [255.0 ("Value") 1.0 ("Value") 5.0 ("Value")] -> w310
              tunnel: [128.0 ("Value") 0.0 ("Value") 0.0 ("Value")] -> w309
              tunnel: [64.0 ("Value") 0.5 ("Value") 1.0 ("Value")] -> w308
              frame "PWM" {
              }
              frame "Motor", Default {
              }
              frame "Analog Out" {
              }
            }
            n184 = property on="Test Slider" class="Slide (strict)"("Visible"=w313) -> ()  [unwired: 2 in, 2 out]
            n185 = property on="Test Ring" class="Ring (strict)"("Visible"=w313) -> ()  [unwired: 2 in, 2 out]
            n186 = property on="On/Off" class="Bool (strict)"("Visible"=w313) -> ()  [unwired: 2 in, 2 out]
            n187 = property on="Rev/Fwd" class="Clust (strict)"("Visible"=w313) -> ()  [unwired: 2 in, 2 out]
            n188 = property on="Motor" class="Clust (strict)"("Visible"=TRUE) -> ()  [unwired: 2 in, 2 out]
            n189 = property on="Value" class="Slide (strict)"("Value"=w309, "Scale.Minimum"=w311, "Scale.Maximum"=w310, "Scale.Increment"=w308) -> ()  [unwired: 2 in, 2 out]
          }
          frame "Servo" {
            w329 = FALSE ("Visible")
            n190 = call <vilib>:"NT Read Number.vi"("Name"=w331) -> ("Numeric"=w330:dbl)  [unwired: 9 in, 1 out]
            n191 = property on="Motor" class="Clust (strict)"("Visible"=w329) -> ()  [unwired: 2 in, 2 out]
            n192 = property on="Test Ring" class="Ring (strict)"("Visible"=w329) -> ()  [unwired: 2 in, 2 out]
            n193 = property on="On/Off" class="Bool (strict)"("Visible"=w329) -> ()  [unwired: 2 in, 2 out]
            n194 = property on="Rev/Fwd" class="Clust (strict)"("Visible"=w329) -> ()  [unwired: 2 in, 2 out]
            n195 = property on="Test Slider" class="Slide (strict)"("Visible"=TRUE, "Scale.Maximum"=170.0 ("Scale.Range:Maximum")) -> ()  [unwired: 2 in, 2 out]
            n196 = local write "Test Slider"(w330) -> ()
          }
          frame "Relay", "Solenoid" {
            w332 = FALSE ("Visible")
            n197 = property on="Motor" class="Clust (strict)"("Visible"=w332) -> ()  [unwired: 2 in, 2 out]
            n198 = property on="Test Slider" class="Slide (strict)"("Visible"=w332) -> ()  [unwired: 2 in, 2 out]
            n199 = property on="Test Ring" class="Ring (strict)"("Visible"=w332) -> ()  [unwired: 2 in, 2 out]
            n200 = Search and Replace String(input string=w333, search string="/Value  **", replace string="/Direction") -> (result string=w339:string)  [unwired: 5 in, 3 out]
            n201 = call <vilib>:"NT Read String.vi"("Name"=w339) -> ("String"=w337:string)  [unwired: 9 in, 1 out]
            n202 = Equal?(x="Both directions", y=w337) -> (x = y?=w335:bool)
            n203 = property on="Rev/Fwd" class="Clust (strict)"("Visible"=w335) -> ()  [unwired: 2 in, 2 out]
            n204 = Not(x=w335) -> (.not. x?=w336:bool)
            n205 = property on="On/Off" class="Bool (strict)"("Visible"=w336, "Caption.Text"=w334) -> ()  [unwired: 2 in, 2 out]
          }
          frame "Compressor", "Digital Out" {
            w342 = FALSE ("Visible")
            # "Get direction and finish"
            n206 = property on="Test Ring" class="Ring (strict)"("Visible"=w342) -> ()  [unwired: 2 in, 2 out]
            n207 = property on="Motor" class="Clust (strict)"("Visible"=w342) -> ()  [unwired: 2 in, 2 out]
            n208 = property on="Test Slider" class="Slide (strict)"("Visible"=w342) -> ()  [unwired: 2 in, 2 out]
            n209 = property on="Rev/Fwd" class="Clust (strict)"("Visible"=FALSE) -> ()  [unwired: 2 in, 2 out]
            n210 = property on="On/Off" class="Bool (strict)"("Visible"=TRUE, "Caption.Text"=w343) -> ()  [unwired: 2 in, 2 out]
          }
          frame "Camera" {
            n211 = call <vilib>:"Get Last Path Segment.vi"("String in"=w350) -> ("String out"=w351:string)  [unwired: 10 in]
            n212 = property on="Rev/Fwd" class="Clust (strict)"("Visible"=FALSE) -> ()  [unwired: 2 in, 2 out]
            n213 = case shown="\"White Balance  **\"" w351 {
              tunnel: w350 -> [w357 w366 w375 w384 w393 _ w399]
              tunnel: w349 -> [w355 w363 w372 w381 w390 _ _]
              frame "Size  **" {
                n214 = Index Array(array=w355) -> (element=w354:cluster{string[]})  [unwired: 1 in]
                n215 = call <vilib>:"NT Read String.vi"("Name"=w357) -> ("String"=w356:string)  [unwired: 9 in, 1 out]
                n216 = property on="Test Ring" class="Ring (strict)"("Visible"=TRUE) -> ()  [unwired: 2 in, 2 out]
                n217 = property on="Test Slider" class="Slide (strict)"("Visible"=FALSE) -> ()  [unwired: 2 in, 2 out]
                n218 = Unbundle(w354) -> (w352:string[])
                n219 = Match First String(2:w352, 3:w356) -> (0:w353:i32)  [unwired: 1 out]
                n220 = property on="Test Ring" class="Ring (strict)"("Value"=w353, "Strings []"=w352) -> ()  [unwired: 2 in, 2 out]
              }
              frame "White Balance  **" {
                n221 = call <vilib>:"NT Read String.vi"("Name"=w366) -> ("String"=w365:string)  [unwired: 9 in, 1 out]
                n222 = Index Array(array=w363, index=1) -> (element=w364:cluster{string[]})
                n223 = property on="Test Ring" class="Ring (strict)"("Visible"=TRUE) -> ()  [unwired: 2 in, 2 out]
                n224 = property on="Test Slider" class="Slide (strict)"("Visible"=FALSE) -> ()  [unwired: 2 in, 2 out]
                n225 = Unbundle(w364) -> (w361:string[])
                n226 = Match First String(2:w361, 3:w365) -> (0:w360:i32)  [unwired: 1 out]
                n227 = property on="Test Ring" class="Ring (strict)"("Value"=w360, "Strings []"=w361) -> ()  [unwired: 2 in, 2 out]
              }
              frame "Exposure  **" {
                n228 = call <vilib>:"NT Read String.vi"("Name"=w375) -> ("String"=w374:string)  [unwired: 9 in, 1 out]
                n229 = Index Array(array=w372, index=2) -> (element=w373:cluster{string[]})
                n230 = property on="Test Ring" class="Ring (strict)"("Visible"=TRUE) -> ()  [unwired: 2 in, 2 out]
                n231 = property on="Test Slider" class="Slide (strict)"("Visible"=FALSE) -> ()  [unwired: 2 in, 2 out]
                n232 = Unbundle(w373) -> (w369:string[])
                n233 = Match First String(2:w369, 3:w374) -> (0:w370:i32)  [unwired: 1 out]
                n234 = property on="Test Ring" class="Ring (strict)"("Value"=w370, "Strings []"=w369) -> ()  [unwired: 2 in, 2 out]
              }
              frame "Exposure Priority  **" {
                n235 = call <vilib>:"NT Read String.vi"("Name"=w384) -> ("String"=w383:string)  [unwired: 9 in, 1 out]
                n236 = Index Array(array=w381, index=3) -> (element=w382:cluster{string[]})
                n237 = property on="Test Ring" class="Ring (strict)"("Visible"=TRUE) -> ()  [unwired: 2 in, 2 out]
                n238 = property on="Test Slider" class="Slide (strict)"("Visible"=FALSE) -> ()  [unwired: 2 in, 2 out]
                n239 = Unbundle(w382) -> (w378:string[])
                n240 = Match First String(2:w378, 3:w383) -> (0:w379:i32)  [unwired: 1 out]
                n241 = property on="Test Ring" class="Ring (strict)"("Value"=w379, "Strings []"=w378) -> ()  [unwired: 2 in, 2 out]
              }
              frame "Color Enable  **" {
                n242 = call <vilib>:"NT Read String.vi"("Name"=w393) -> ("String"=w392:string)  [unwired: 9 in, 1 out]
                n243 = Index Array(array=w390, index=4) -> (element=w391:cluster{string[]})
                n244 = property on="Test Ring" class="Ring (strict)"("Visible"=TRUE) -> ()  [unwired: 2 in, 2 out]
                n245 = property on="Test Slider" class="Slide (strict)"("Visible"=FALSE) -> ()  [unwired: 2 in, 2 out]
                n246 = Unbundle(w391) -> (w387:string[])
                n247 = Match First String(2:w387, 3:w392) -> (0:w388:i32)  [unwired: 1 out]
                n248 = property on="Test Ring" class="Ring (strict)"("Value"=w388, "Strings []"=w387) -> ()  [unwired: 2 in, 2 out]
              }
              frame Default {
                n249 = property on="Test Slider" class="Slide (strict)"("Visible"=FALSE) -> ()  [unwired: 2 in, 2 out]
                n250 = property on="Test Ring" class="Ring (strict)"("Visible"=FALSE) -> ()  [unwired: 2 in, 2 out]
              }
              frame "Brightness  **", "Color Level  **", "Compression  **", "FPS  **", "Sharpness  **" {
                n251 = call <vilib>:"NT Read Number.vi"("Name"=w399) -> ("Numeric"=w398:dbl)  [unwired: 9 in, 1 out]
                n252 = property on="Test Ring" class="Ring (strict)"("Visible"=FALSE) -> ()  [unwired: 2 in, 2 out]
                n253 = property on="Test Slider" class="Slide (strict)"("Visible"=TRUE, "Scale.Maximum"=100.0 ("Scale.Range:Maximum")) -> ()  [unwired: 2 in, 2 out]
                n254 = local write "Test Slider"(w398) -> ()
              }
            }
            n255 = property on="Motor" class="Clust (strict)"("Visible"=FALSE) -> ()  [unwired: 2 in, 2 out]
            n256 = property on="On/Off" class="Bool (strict)"("Visible"=FALSE) -> ()  [unwired: 2 in, 2 out]
          }
        }
      }
      event "Test Name": Mouse Enter {
        # "Populate the ring with the list of tests"
        n257 = event-data() -> ()  [unwired: 1 in, 1 out]
        n258 = call <vilib>:"NT Read String Array.vi"("Name"="/TestMode/TestList") -> ("String Array"=w408:string[])  [unwired: 9 in, 1 out]
        n259 = Build Array (concatenate)("Select the test to run...", w408) -> (w407:string[])
        n260 = property on="Test Name" class="Ring (strict)"("Strings []"=w407) -> ()  [unwired: 2 in, 2 out]
      }
      event "Test Name": Value Change {
        w411 = FALSE ("Visible")
        # "Tell the robot the test name to run"
        n261 = event-data() -> ("NewVal"=w415:u16)  [unwired: 1 in]
        n262 = property on="Test Name" class="Ring (strict)"() -> ("Strings []"=w416:string[])  [unwired: 2 in, 2 out]
        n263 = property on="Test Ring" class="Ring (strict)"("Visible"=w411) -> ()  [unwired: 2 in, 2 out]
        n264 = property on="Motor" class="Clust (strict)"("Visible"=w411) -> ()  [unwired: 2 in, 2 out]
        n265 = property on="Test Slider" class="Slide (strict)"("Visible"=w411) -> ()  [unwired: 2 in, 2 out]
        n266 = property on="On/Off" class="Bool (strict)"("Visible"=w411) -> ()  [unwired: 2 in, 2 out]
        n267 = property on="Rev/Fwd" class="Clust (strict)"("Visible"=w411) -> ()  [unwired: 2 in, 2 out]
        n268 = local write "Progress"(T5 {"Test Progress"=0, "Test Progress Text"=""} ("Progress")) -> ()
        n269 = property on="Progress" class="Clust (strict)"("Visible"=TRUE) -> ()  [unwired: 2 in, 2 out]
        n270 = Index Array(array=w416, index=w415) -> (element=w414:string)
        n271 = call <vilib>:"NT Write String.vi"("String"=w414, "Name"="/TestMode/TestName") -> ()  [unwired: 9 in, 1 out]
      }
      event "Position Selector": Mouse Enter {
        # "Populate the combo box with the list of autonomous options"
        n272 = event-data() -> ()  [unwired: 1 in, 1 out]
        n273 = call <vilib>:"NT Read String Array.vi"("Name"="Auto List") -> ()  [unwired: 9 in, 2 out]
      }
      event "Position Selector": Value Change {
        # "User modified the Auto Selection. Write to NT variable so robot knows."
        n274 = event-data() -> ()  [unwired: 1 in, 1 out]
        n275 = call <vilib>:"NT Write String.vi"("Name"="Auto Selector") -> ()  [unwired: 10 in, 1 out]
      }
      event "Command Selection": Value Change {
        # "Get the params and show in table"
        n276 = event-data() -> ("NewVal"=w427:i32)  [unwired: 1 in]
        n277 = property on="Command Selection" class="MCListbox (strict)"() -> ("ItemNames"=w425:string[][])  [unwired: 2 in, 2 out]
        n278 = call <vilib>:"WPI_DashboardUpdate Command Params.vi"("NewVal"=w427, "Commands"=w425, "Param Tbl"=w426) -> ()  [unwired: 8 in, 1 out]
      }
      event "Execute Command": Value Change {
        # "Started one, Unique ID holds\nresponse"
        n279 = event-data() -> ()  [unwired: 1 in, 1 out]
        n280 = property on="Command Selection" class="MCListbox (strict)"() -> ("ItemNames"=w439:string[][])  [unwired: 2 in, 2 out]
        n281 = Index Array(array=w439, index (row)="Command Selection", index (col)=0) -> (element=w437:string)
        n282 = call <vilib>:"Invoke Commands.vi"("Command Params"="Command Params", "Function Name"=w437) -> ("Params"=w433:u8, "Started"=w432:bool)  [unwired: 7 in, 1 out]
        n283 = Array Subset(array="Command Params", length (row)=w433) -> (w434:string[][])  [unwired: 3 in]
        n284 = Select(t="Executing" ("Cmd Status"), s=w432, f="" ("Cmd Status")) -> (s? t:f=→"Cmd Status":string)
      }
      event "Command Selection": Double Click {
        n285 = event-data() -> ("Row"=w449:i32)  [unwired: 1 in]
        n286 = property on="Command Selection" class="MCListbox (strict)"() -> ("ItemNames"=w452:string[][])  [unwired: 2 in, 2 out]
        n287 = local read "Command Params"() -> (w447:string[][])
        n288 = Index Array(array=w452, index (row)=w449, index (col)=0) -> (element=w450:string)
        n289 = call <vilib>:"Invoke Commands.vi"("Command Params"=w447, "Function Name"=w450) -> ("Params"=w446:u8, "Started"=w441:bool)  [unwired: 7 in, 1 out]
        n290 = Array Subset(array=w447, length (row)=w446) -> (w445:string[][])  [unwired: 3 in]
        n291 = Select(t="Executing" ("Cmd Status"), s=w441, f="" ("Cmd Status")) -> (s? t:f=w442:string)
        n292 = local write "Cmd Status"(w442) -> ()
      }
      event "CheckList": Double Click {
        # "Shift clears all"
        # "Update symbols on the listbox"
        n293 = event-data() -> ("PlatMods.Shift"=w455:bool, "Row"=w457:i32)  [unwired: 1 in]
        n294 = case shown="True" w455 {
          tunnel: w457 -> [w461 _]
          tunnel: 1 -> [w460 _]
          frame False {
            n295 = property on="CheckList" class="LstBox (strict)"() -> ("Item Symbols"=w459:i32[])  [unwired: 2 in, 2 out]
            n296 = Replace Array Subset(array=w459, new element=w460, index=w461) -> (w458:i32[])
            n297 = property on="CheckList" class="LstBox (strict)"("Item Symbols"=w458) -> ()  [unwired: 2 in, 2 out]
          }
          frame True {
            w462 = 0 ("Top Row")
            n298 = property on="CheckList" class="LstBox (strict)"() -> ("Number of Rows"=w464:u32)  [unwired: 2 in, 2 out]
            n299 = Initialize Array(0, w464) -> (w463:i32[])
            n300 = property on="CheckList" class="LstBox (strict)"("Top Row"=w462, "Value"=w462, "Item Symbols"=w463) -> ()  [unwired: 2 in, 2 out]
          }
        }
      }
      event "CheckList": Key Down {
        # "Update symbols on the listbox\nLeft and right keys check and uncheck"
        n301 = event-data() -> ("VKey"=w469:T13)  [unwired: 1 in]
        n302 = case shown="\"Left\", \"Right\"" w469 {
          selector: w469 -> [w474 _]
          tunnel: eventvkey."Left" ("VKey") -> [w472 _]
          frame "Left", "Right" {
            n303 = Equal?(x=w472, y=w474) -> (x = y?=w473:bool)
            n304 = Select(t=0, s=w473, f=1) -> (s? t:f=w475:i32)
            n305 = property on="CheckList" class="LstBox (strict)"() -> ("Item Symbols"=w478:i32[])  [unwired: 2 in, 2 out]
            n306 = Replace Array Subset(array=w478, new element=w475, index="CheckList") -> (w477:i32[])
            n307 = property on="CheckList" class="LstBox (strict)"("Item Symbols"=w477) -> ()  [unwired: 2 in, 2 out]
          }
          frame Default {
          }
        }
      }
      event "DB Camera Config": Value Change {
        # "Show or hide the cluster of controls, store in ini file"
        n308 = event-data() -> ("NewVal"=w483:bool)  [unwired: 1 in]
        n309 = case shown="False" w483 {
          tunnel: w482 -> [w492 _]
          tunnel: [w485 w503] -> w481
          tunnel: w480 -> [w484 w503]
          frame False {
            w499 = "Camera"
            w502 = FALSE ("Visible")
            n310 = Index Array(array=w492) -> (element=w495:cluster{string[]})  [unwired: 1 in]
            n311 = local write "DB Camera Config"(w502) -> ()
            n312 = property on="Camera Settings" class="Clust (strict)"("Visible"=w502) -> ()  [unwired: 2 in, 2 out]
            n313 = Unbundle(w495) -> (w494:string[])
            n314 = local read "Camera Settings"() -> (w491:T2)
            n315 = Unbundle(w491) -> ("Frame Rate"=w490:i32, "Compression"=w489:i32, "Size"=w493:u16)
            n316 = Index Array(array=w494, index=w493) -> (element=w488:string)
            n317 = call-poly <vilib>:"Write Key.vi"("section"=w499, "value"=w488, "key"="Size", "refnum"=w484) -> ("refnum out"=w501:T11)  [unwired: 2 in, 5 out]
            n318 = call-poly <vilib>:"Write Key.vi"("section"=w499, "value"=w490, "key"="FrameRate", "refnum"=w501) -> ("refnum out"=w500:T11)  [unwired: 1 in, 6 out]
            n319 = call-poly <vilib>:"Write Key.vi"("section"=w499, "value"=w489, "key"="Compression", "refnum"=w500) -> ("refnum out"=w486:T11)  [unwired: 1 in, 6 out]
            n320 = call <vilib>:"Close Config Data.vi"("refnum"=w486) -> ("file path"=w487:path)  [unwired: 2 in, 8 out]
            n321 = call <vilib>:"Open Config Data.vi"("configuration file path"=w487) -> ("refnum"=w485:T11)  [unwired: 8 in, 2 out]
          }
          frame True {
            n322 = property on="Camera Settings" class="Clust (strict)"("Visible"=TRUE) -> ()  [unwired: 2 in, 2 out]
          }
        }
      }
      event "Camera Settings": Value Change {
        # "Update summary string when any elements of DB camera change"
        n323 = event-data() -> ("NewVal"=w517:T2)  [unwired: 1 in]
        n324 = Index Array(array=w513) -> (element=w512:cluster{string[]})  [unwired: 1 in]
        n325 = Unbundle(w517) -> ("Frame Rate"=w508:i32, "Compression"=w507:i32, "Size"=w510:u16)
        n326 = Unbundle(w512) -> (w511:string[])
        n327 = Index Array(array=w511, index=w510) -> (element=w509:string)
        n328 = Format Into String(format string="%s   %dfps   %d%%", w509, w508, w507) -> (resulting string=w514:string)  [unwired: 2 in, 1 out]
        n329 = Build Array(w514) -> (w515:string[])
        n330 = property on="DB Camera Config" class="Bool (strict)"("Strings [4]"=w515) -> ()  [unwired: 2 in, 2 out]
      }
      event "Motor.Enable": Value Change {
        # "When the test mode otor enable helper is set, update that\ntree row item's value"
        n331 = event-data() -> ("NewVal"=w524:bool)  [unwired: 1 in]
        n332 = Unbundle("Motor") -> ("Value"=w523:dbl)  [unwired: 1 out]
        n333 = Select(t=w523, s=w524, f=0.0) -> (s? t:f=w521:dbl)
        n334 = call <vilib>:"NT Write Number.vi"("Numeric"=w521, "Name"=w520) -> ()  [unwired: 9 in, 1 out]
      }
      event "Test Slider": Value Change {
        # "When the test mode slider helper is set, update that\ntree row item's value"
        n335 = event-data() -> ("NewVal"=w528:dbl)  [unwired: 1 in]
        n336 = call <vilib>:"NT Write Number.vi"("Numeric"=w528, "Name"=w529) -> ()  [unwired: 9 in, 1 out]
      }
      event "On/Off": Value Change {
        # "When the test mode on/off helper value is set, update that\ntree row item's value"
        n337 = event-data() -> ("NewVal"=w534:bool)  [unwired: 1 in]
        n338 = Boolean To (0,1)(Boolean=w534) -> (0, 1=w533:i16)
        n339 = call <vilib>:"NT Write Number.vi"("Numeric"=w533, "Name"=w532) -> ()  [unwired: 9 in, 1 out]
      }
      event "Rev/Fwd": Value Change {
        # "When the test mode helper value for relays is set, update that\ntree row item's value"
        n340 = event-data() -> ("NewVal.Forward"=w543:bool, "NewVal.Reverse"=w542:bool)  [unwired: 1 in]
        n341 = Boolean To (0,1)(Boolean=w543) -> (0, 1=w539:i16)
        n342 = Boolean To (0,1)(Boolean=w542) -> (0, 1=w541:i16)
        n343 = Negate(x=w541) -> (-x=w540:i16)
        n344 = Add(x=w539, y=w540) -> (x+y=w538:i16)
        n345 = call <vilib>:"NT Write Number.vi"("Numeric"=w538, "Name"=w537) -> ()  [unwired: 9 in, 1 out]
      }
      event "Test Ring": Value Change {
        # "When a test mode helper value is selected from the ring,\nset the tree item's variable to the string value"
        n346 = event-data() -> ("NewVal"=w548:u16)  [unwired: 1 in]
        n347 = property on="Test Ring" class="Ring (strict)"() -> ("Strings []"=w549:string[])  [unwired: 2 in, 2 out]
        n348 = Index Array(array=w549, index=w548) -> (element=w547:string)
        n349 = call <vilib>:"NT Write String.vi"("String"=w547, "Name"=w546) -> ()  [unwired: 9 in, 1 out]
      }
      event "Rec Mode": Value Change {
        # "Update globals for recording mode and path to read log from.\nClear when logging and let NetworkTables set path for vision to\nuse."
        n350 = event-data() -> ("NewVal"=w561:enum32{"Stop", "Record", "Playback"})  [unwired: 1 in]
        n351 = global write "WPI_DashboardLogging Global.vi" "Logging Filename"(path "") -> ()
        n352 = global write "WPI_DashboardLogging Global.vi" "Recording"(w561) -> ()
        n353 = case shown="\"Playback\"" w561 {
          tunnel: w560 -> [_ w563 w572]
          tunnel: [_ _ w571] -> w557
          tunnel: [_ _ w570] -> _
          tunnel: w555 -> [_ _ w568]
          tunnel: cluster{i32, i32} {-250, 170} -> [_ _ w567]
          tunnel: [_ _ T14 {"Image Size"=TRUE, "Image Type"=TRUE, "Pixel Value"=TRUE, "ROI Information"=TRUE, "Zoom Factor"=FALSE} ("Image Information Shown:All Elements")] -> w553
          tunnel: [_ _ TRUE ("Zoom Factor")] -> w552
          tunnel: w551 -> [_ _ w564]
          frame Default {
          }
          frame "Stop", "Record" {
            # "Place Window too"
            n354 = invoke class="VI" method="FP.Close"(reference=w563) -> (reference out=w562:refnum<vi>)  [unwired: 2 in, 2 out]
            n355 = invoke class="VI" method="Abort VI"(reference=w562) -> ()  [unwired: 2 in, 3 out]
          }
          frame "Playback" {
            n356 = call "Open Playback Panel.vi"("Offset"=w567, "DB VI Ref"=w568, "Playback in"=w572) -> ("Playback out"=w569:refnum<vi>)  [unwired: 8 in]
            n357 = register-events(w569, w564) -> (reference out=w571:refnum<event-registration>, error out=w570:errorcluster)  [unwired: 2 in]
          }
        }
        n358 = property on="Camera Image" class="ImageControl"("Image Information Shown"=w553, "Image Information Visible"=w552) -> ()  [unwired: 2 in, 2 out]
        n359 = call <vilib>:"WPI_DashboardNT Log FieldName Cache.vi"("Operation"=enum16{"Lookup/Add", "Index", "Clear"}."Clear") -> ()  [unwired: 8 in, 3 out]
      }
      event Panel Close {
        w574 = enum32{"Stop", "Record", "Playback"}."Stop" ("Rec Mode")
        # "Playback window has been closed, abort"
        n360 = event-data() -> ()  [unwired: 1 in, 4 out]
        n361 = local write "Rec Mode"(w574) -> ()
        n362 = global write "WPI_DashboardLogging Global.vi" "Recording"(w574) -> ()
      }
      event Panel Close {
        # "Abort playback window and ourself"
        n363 = event-data() -> ()  [unwired: 1 in, 4 out]
        n364 = invoke class="VI" method="FP.Close"(reference=w580) -> (reference out=w579:refnum<vi>)  [unwired: 2 in, 2 out]
        n365 = invoke class="VI" method="Abort VI"(reference=w579) -> (error out=w578:errorcluster)  [unwired: 2 in, 2 out]
        n366 = invoke class="VI" method="Abort VI"(error in=w578) -> ()  [unwired: 2 in, 3 out]
      }
      event User Event {
        n367 = event-data() -> ("IDs"=w588:cluster{"RPC field ID":u16, "Unique ID":u16}, "String"=w587:string)  [unwired: 1 in]
        n368 = local write "Cmd Status"("" ("Cmd Status")) -> ()
        n369 = Bundle("IDs"=w588, "String"=w587) -> (w586:T8)  [unwired: 1 in]
        n370 = call <vilib>:"Retrieve RPC Response.vi"("RPC Response"=w586) -> ("Output"=w583:string[][])  [unwired: 10 in]
        n371 = Build Array (concatenate)(w581, w583) -> (w582:string[][])
        n372 = local write "Command Params"(w582) -> ()
      }
      event "Vision": Value Change {
        # "Enable/Disable Compression slider.\nHW USB is hard-coded into the camera"
        n373 = event-data() -> ("NewVal"=w595:u16)  [unwired: 1 in]
        n374 = Equal?(x=w595, y=u32 2 ("milliseconds to wait")) -> (x = y?=w593:bool)
        n375 = Select(t=T15."Disabled and Grayed Out" ("Disabled"), s=w593, f=T15."Enabled" ("Disabled")) -> (s? t:f=w590:T15)
        n376 = property on="Compression" class="Slide (strict)"("DisabledEnum"=w590) -> ()  [unwired: 2 in, 2 out]
      }
      event "Tree": Double Click {
        n377 = event-data() -> ("PlatMods"=w600:T18, "Tag"=w599:string)  [unwired: 1 in]
        n378 = Unbundle(w600) -> ("Shift"=w598:bool)  [unwired: 4 out]
        n379 = Not(x=w598) -> (.not. x?=w597:bool)
        n380 = call <vilib>:"NT Update Persistence.vi"("Persistence"=w597, "Name"=w599) -> ()  [unwired: 9 in, 1 out]
      }
    }
  }
  n381 = call "Adjust Dashboard Window.vi"("Sizing Refnums"=w43, "Size Constraints"=w47, "VI"=w56, "WIn Mode"=w28) -> ()  [unwired: 8 in]
  n382 = Build Array (concatenate)(w29, w54) -> (w53:refnum<vi>[])
  n383 = Obtain Notifier(name (unnamed)="Robot IP Update", notification data type="IP Addr" ("name (unnamed)")) -> (notifier out=w30:refnum<notifier>)  [unwired: 2 in, 2 out]
  n384 = while {
    tunnel: [w614] -> _
    tunnel: w30 -> [w608]
    tunnel: w29 -> [w607]
    tunnel: w28 -> [w603]
    i -> [w614]
    stop <- FALSE stop-if-true
    n385 = call <vilib>:"WPI_DashboardUpdateNames.vi"("Controls on Tab"=w607) -> ()  [unwired: 11 in]
    n386 = local read "Vision"() -> (w605:u16)
    n387 = call <vilib>:"WPI_DashboardRetrieveStatusInfo.vi"("Vision"=w605, "Binding Refnum"=w608, "Window Mode Notifier"=w603, "TCP Cnx"="TCP") -> ("Power and Errors"=w609:T19, "Robot Metrics"=w612:T20, "Status Info"=w613:T21, "Control Info"=w610:T22, "Robot Mode"=w606:T4, "Process?"=w611:bool)  [unwired: 2 in]
    "Mode" <- w606
    n388 = case shown="True" w611 {
      tunnel: w613 -> [_ w630]
      tunnel: w612 -> [_ w629]
      tunnel: w610 -> [_ w628]
      tunnel: w609 -> [_ w627]
      tunnel: w606 -> [_ _]
      frame False {
        n389 = Wait (ms)(milliseconds to wait=u32 20) -> ()  [unwired: 1 out]
      }
      frame True {
        n390 = Unbundle By Name(w628) -> ("Joystick Values"=w626:T23)  [unwired: 1 out]
        n391 = Unbundle By Name(w629) -> ()  [unwired: 1 out]
        n392 = Unbundle By Name(w627) -> ("Camera Addr"=→"Camera IP":string)  [unwired: 1 out]
        n393 = Unbundle By Name(w630) -> ()  [unwired: 2 out]
        n394 = Index Array(array=w626) -> (element #1=w625:T24, element #2=w620:T24)  [unwired: 2 in]
        n395 = call "Prepare Joystick Data for Displays.vi"("Joystick Values"=w625) -> ("Buttons"=→"JS1 Buttons":T25, "Z Axis"=→"JS1 Z":dbl, "Cartesian Data"=→"JS1 Graph":cluster{"X axis":dbl, "X axis":dbl}[])  [unwired: 8 in]
        n396 = call "Prepare Joystick Data for Displays.vi"("Joystick Values"=w620) -> ("Buttons"=→"JS2 Buttons":T25, "Z Axis"=→"JS2 Z":dbl, "Cartesian Data"=→"JS2 Graph":cluster{"X axis":dbl, "X axis":dbl}[])  [unwired: 8 in]
      }
    }
  }
  n397 = while {
    tunnel: w53 -> [w643]
    tunnel: w30 -> [w641]
    tunnel: [w639] -> _
    tunnel: u32 1000 ("milliseconds to wait") -> [w638]
    tunnel: w19 -> [w631]
    i -> [w639]
    stop <- FALSE stop-if-true
    n398 = Wait on Notification(notifier=w641, timeout in ms (-1)=w638) -> (notification=w640:string, timed out?=w636:bool)  [unwired: 2 in, 2 out]
    n399 = local read "Rec Mode"() -> (w634:enum32{"Stop", "Record", "Playback"})
    n400 = Equal?(x=w634, y=u16 2 ("Rec Mode")) -> (x = y?=w635:bool)
    n401 = Compound Arithmetic op=OR(invert w636, w635) -> (w637:bool)
    n402 = case shown="True" w637 {
      tunnel: w643 -> [_ w647]
      tunnel: w640 -> [_ w646]
      tunnel: "Dashboard" -> [_ w645]
      tunnel: w631 -> [_ w644]
      frame False {
      }
      frame True {
        n403 = call <vilib>:"Bind Controls to SmartDashboard.vi"("RPC ref"=w644, "Client Name"=w645, "Bound Control Refs"=w647, "Server IP Address"=w646) -> ()  [unwired: 8 in]
      }
    }
  }
